vi "Out.vi"(8 "错误输入":errorcluster caption="错误输入（无错误）", 10 "超时毫秒(-1)":i32, 11 "队列":refnum<queue>) -> (0 "错误输出":errorcluster, 1 "数据":variant, 2 "指令":string, 3 "队列输出":refnum<queue>)   [LabVIEW 2018]
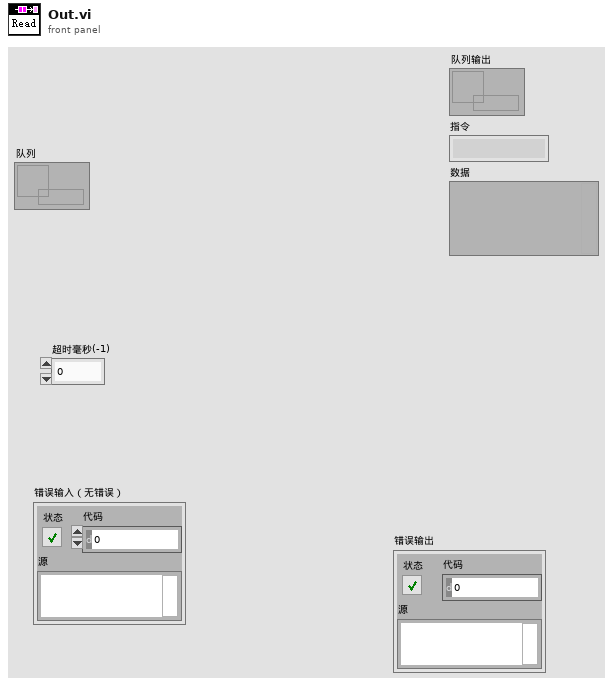
[diagram p1: front panel]
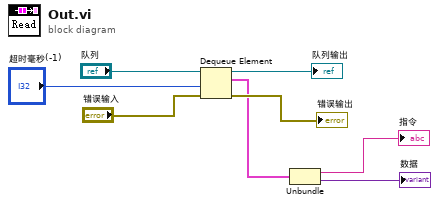
[diagram p0: block diagram]
diagram:
  n1 = Dequeue Element(queue="队列", timeout in ms (-1)="超时毫秒(-1)", error in (no error)="错误输入") -> (queue out=→"队列输出":refnum<queue>, element=w4:cluster{"指令":string, "数据":variant}, error out=→"错误输出":errorcluster)  [unwired: 1 out]
  n2 = Unbundle(w4) -> ("指令"=→"指令":string, "数据"=→"数据":variant)
